vi "strerror.vi"(7 "path override":path, 8 "error in (no error)":errorcluster, 11 "errnum_":i32) -> (0 "error out":errorcluster, 3 "function return":string)   [LabVIEW 2025, in "LibZMQ.lvlib"]
doc: "ZMQ_EXPORT const char *zmq_strerror (int errnum_);"
uses:
  LibZMQ.lvlib
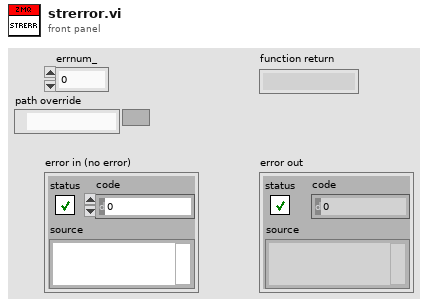
[diagram p1: front panel]
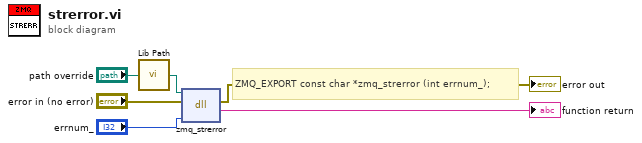
[diagram p0: block diagram]
diagram:
  # "ZMQ_EXPORT const char *zmq_strerror (int errnum_);"
  n1 = call "Lib Path.vi"("path override"="path override") -> ("lib path"=w2:path)
  n2 = dll-call lib="home/james/Documents/ZeroMQ_LV/libzmq-v143-mt-4_3_6/libzmq.so" fn="zmq_strerror"(path in=w2, error in="error in (no error)", "errnum_"="errnum_") -> (error out=→"error out":errorcluster, "return type"=→"function return":string)  [unwired: 2 in, 1 out]
